vi "Control - Generic - Intake Air Measured Host.vi"() -> ()   [LabVIEW 2015, in "ECS-Host.lvlib"]
uses:
  ECS-Host.lvlib
  <vilib>/addons/Software Calibration Management/XControls/TBL2D.xctl
  <vilib>/addons/Software Calibration Management/XControls/TBL1D.xctl
  Typedefs/MISC/Intake Charge Mode.ctl
  ECS-Shared.lvlib
panel:
  out "VE_Calc":sgl caption="[]"
  in  "_MAF Only Tab Control":enum32{"MAF Only"}(tab)
  out "AirflowNoEGR_Calc":sgl caption="[kg/hr]"
  out "AirflowCorr_Calc":sgl caption="[]"
  in  "AirflowECTCorr_Tbl":cluster{"X":sgl[], "Y":sgl[]}(xcontrol)
  in  "AirflowCorr_Tbl":cluster{"X":sgl[], "Y":sgl[], "Z":sgl[][]}(xcontrol) caption="[]"
  out "AirflowNoEGR_TblOut":sgl caption="[]"
  in  "AirflowNoEGR_Tbl":cluster{"X":sgl[], "Y":sgl[], "Z":sgl[][]}(xcontrol) caption="[]"
  in  "AirflowCorr_E":bool
  in  "_VE Tab Control":enum32{"VE Table", "VE Learn Table"}(tab)
  out "VE_TblOut":sgl caption="[]"
  in  "VE_Tbl":cluster{"X":sgl[], "Y":sgl[], "Z":sgl[][]}(xcontrol) caption="[]"
  in  "VELearn_E":bool
  in  "VELearnGain":sgl
  in  "VELearn_Tbl":cluster{"X":sgl[], "Y":sgl[], "Z":sgl[][]}(xcontrol)
  out "PrevFuel":sgl caption="[]"
  in  "EGRMassFlow_PreCalcE":bool
  out "EGRMassFlow_PreCalc":sgl caption="[]"
  out "ConservationOfMassFault":bool
  out "ConservationOfMassError":sgl caption="[]"
  out "AvailableAirMassFlow":sgl caption="[]"
  out "AvailableAirMass":sgl caption="[]"
  out "ChargeAirMassFlow":sgl caption="[]"
  out "ChargeAirMass":sgl caption="[]"
  out "EGRMassFlow":sgl caption="[]"
  out "EGRMass":sgl caption="[]"
  out "PrevLambda":sgl caption="[]"
  out "FreshAirMassFlow":sgl caption="[]"
  out "FreshAirMass":sgl caption="[]"
  out "IntakeMAT":sgl caption="[]"
  out "IntakeMAP":sgl caption="[]"
  out "MAF":sgl caption="[kg/hr]"
  out "EngineSpeed":sgl caption="[]"
  in  "IntakeChargeMode":T1
  # "Measured Values"
  # "MAF Only (No EGR):\nEGR Flow (kg/hr) = 0\nMAF Only (EGR):\nEGR Flow (kg/hr)  =  Airflow_NoEGR - Intake Air\nMAP Only (No EGR):\nEGR Flow (kg/hr) = 0\nMAP Only (EGR):\nEGR Flow (kg/hr)  =  Pre-Calc EGR Flow\nMAF + MAP (EGR):\nEGR Flow (kg/hr)  =  Charge Air - Intake Air"
  # "Select 'MAP' related mode for additional controls"
  # "Calculated Values"
  # "Select 'MAF Only' mode for additional controls"
  # "+"
  # "="
  # "x"
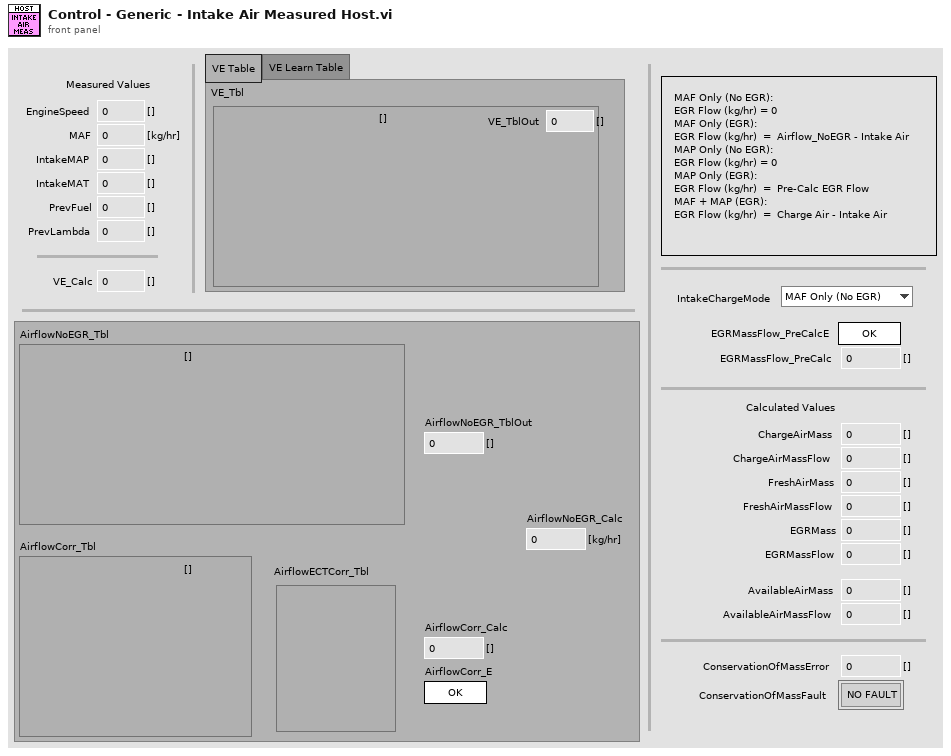
[diagram p1: front panel]
types:
  T1 = typedef "ECS-Shared.lvlib/Intake Charge Mode.ctl" = enum32{"MAF Only (No EGR)", "MAF Only (EGR)", "MAP Only (No EGR)", "MAP Only (EGR)", "MAF + MAP (EGR)"}
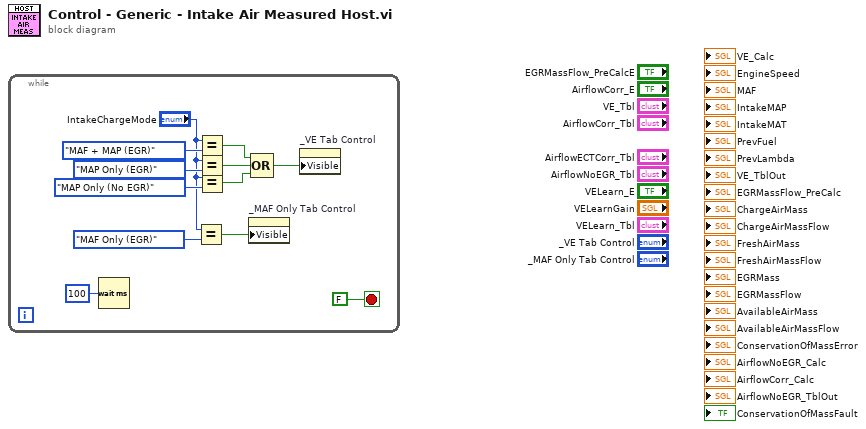
[diagram p0: block diagram]
diagram:
  n1 = while {
    stop <- FALSE stop-if-true
    n2 = Wait (ms)(milliseconds to wait=u32 100) -> ()  [unwired: 1 out]
    n3 = Equal?(x="IntakeChargeMode", y=Intake_Charge_Mode."MAF Only (EGR)" ("Intake Charge Mode")) -> (x = y?=w1:bool)
    n4 = Equal?(x="IntakeChargeMode", y=Intake_Charge_Mode."MAF + MAP (EGR)" ("Intake Charge Mode")) -> (x = y?=w7:bool)
    n5 = Equal?(x="IntakeChargeMode", y=Intake_Charge_Mode."MAP Only (EGR)" ("Intake Charge Mode")) -> (x = y?=w6:bool)
    n6 = Equal?(x="IntakeChargeMode", y=Intake_Charge_Mode."MAP Only (No EGR)" ("Intake Charge Mode")) -> (x = y?=w5:bool)
    n7 = property on="_MAF Only Tab Control" class="TabCtl (strict)"("Visible"=w1) -> ()  [unwired: 2 in, 2 out]
    n8 = Compound Arithmetic op=OR(w7, w6, w5) -> (w4:bool)
    n9 = property on="_VE Tab Control" class="TabCtl (strict)"("Visible"=w4) -> ()  [unwired: 2 in, 2 out]
  }
